vi "Begin.vi"(8 "error in":errorcluster) -> (0 "error out":errorcluster)   [LabVIEW 2019]
doc: "Called before other user functions, this VI is expected to open initial I/O refnums, load in file data, and do all program initialization. Notice that the <B>error out</B> terminal is simply used for data flow. Wiring it to other structures or subVIs ensures that this VI runs first."
uses:
  <vilib>/Rock Robotics/WPI/DriverStation/WPI_DriverStationRobotMode2.ctl
  <vilib>/Rock Robotics/WPI/Joystick/WPI_JoystickDeviceEnum.ctl
  <vilib>/Rock Robotics/SystemInterfaces/DIO/FPGA_DIOChannel.ctl
  <vilib>/Rock Robotics/WPI/ThirdParty/REV Robotics/SPARK MAX/Typedef/Spark MAX Idle Mode.ctl
  <vilib>/Rock Robotics/WPI/ThirdParty/REV Robotics/SPARK MAX/Typedef/Spark MAX Motor Type.ctl
  <vilib>/Rock Robotics/WPI/SafetyOutput/WPI_SafetyOutputConfigMenu.ctl
  <vilib>/Rock Robotics/WPI/Solenoid/WPI_SolenoidChannel.ctl
  <vilib>/Rock Robotics/WPI/Encoder/WPI_EncoderType.ctl
  <vilib>/Rock Robotics/SystemInterfaces/DIO/FPGA_DIORelayChannel.ctl
  <vilib>/Rock Robotics/WPI/Relay/WPI_RelayDirection.ctl
  <vilib>/Rock Robotics/WPI/ThirdParty/Phoenix-LabVIEW/Motor Controller/Controls/CTRE_Phoenix_MotorControl_ControlMode.ctl
  Robot Global Data.vi
  <vilib>/Rock Robotics/Network Tables/NT Write String Array.vi
  <vilib>/Rock Robotics/WPI/Counter/WPI_CounterDigitalInputToDigitalSource.vi
  <vilib>/Rock Robotics/WPI/RobotDrive/WPI_RobotDriveOpen4MotorWithExistingMotors.vi
  <vilib>/Rock Robotics/WPI/Solenoid/WPI_SolenoidOpenDouble.vi
  <vilib>/Rock Robotics/WPI/Switch/WPI_SwitchOpenLimit.vi
  <vilib>/Rock Robotics/WPI/Utilities/WPI_GetSetVariantRefNum.vi
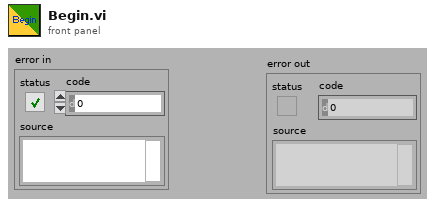
[diagram p1: front panel]
types:
  T1 = typedef "CTRE_Phoenix_MotorControl_ControlMode.ctl" = u16
  T2 = typedef "WPI_RelayDirection.ctl" = enum16{"Both directions", "Forward only", "Reverse only"}
  T3 = typedef "FPGA_DIORelayChannel.ctl" = enum8{"Relay 0", "Relay 1", "Relay 2", "Relay 3", "Invalid"}
  T4 = typedef "WPI_SolenoidChannel.ctl" = enum8{"Solenoid 0", "Solenoid 1", "Solenoid 2", "Solenoid 3", "Solenoid 4", "Solenoid 5", "Solenoid 6", "Solenoid 7", "Invalid"}
  T5 = typedef "WPI_EncoderType.ctl" = enum16{"1x", "2x", "4x"}
  T6 = typedef "FPGA_DIOChannel.ctl" = enum8{"DIO 0", "DIO 1", "DIO 2", "DIO 3", "DIO 4", "DIO 5", "DIO 6", "DIO 7", "DIO 8", "DIO 9", "DIO MXP 0", "DIO MXP 1", "DIO MXP 2", "DIO MXP 3", "DIO MXP 4", "DIO MXP 5", "DIO MXP 6", "DIO MXP 7", "DIO MXP 8", "DIO MXP 9", "DIO MXP 10", "DIO MXP 11", "DIO MXP 12", "DIO MXP 13", "DIO MXP 14", "DIO MXP 15", "SPI Port CS1", "SPI Port CS2", "SPI Port CS3", "SPI Port MISO", "SPI Port MOSI", "Invalid"}
  T7 = typedef "WPI_SafetyOutputConfigMenu.ctl" = enum16{"Enable", "Disable"}
  T8 = typedef "Spark MAX Idle Mode.ctl" = enum16{"Coast", "Brake"}
  T9 = typedef "Spark MAX Motor Type.ctl" = enum16{"Brushed", "Brushless"}
  T10 = typedef "WPI_JoystickDeviceEnum.ctl" = enum16{"USB 0", "USB 1", "USB 2", "USB 3", "USB 4", "USB 5"}
  T11 = typedef "WPI_DriverStationRobotMode2.ctl" = enum16{"Autonomous Disabled", "Autonomous Enabled", "Teleop Disabled", "Teleop Enabled", "Disconnected", "Finish", "Test Disabled", "Test Enabled", "Emergency Stopped"}
  T12 = typedef "WPI_MotorControlDeviceRef.ctl" = cluster{"DeviceStatus":errorcluster, "Type":T13, "PWM":cluster{"PWM Channel":T14, "DeadBand":T15}, "CAN":cluster{"Device Number":u8, "SetOutput VI Ref":variant, "GetOutput VI Ref":variant, "Enable VI Ref":variant, "Disable VI Ref":variant, "Data":variant}, "Invert":bool, "DIO PWM":cluster{"PWM \"Enable\" Channel":T14, "DIOChannel":T6, "PWM Rate":dbl}}
  T13 = typedef "WPI_MotorControlType.ctl" = enum16{"PWM", "CAN", "DIO PWM"}
  T14 = typedef "FPGA_DIOPWMChannel.ctl" = enum8{"PWM 0", "PWM 1", "PWM 2", "PWM 3", "PWM 4", "PWM 5", "PWM 6", "PWM 7", "PWM 8", "PWM 9", "PWM MXP 0", "PWM MXP 1", "PWM MXP 2", "PWM MXP 3", "PWM MXP 4", "PWM MXP 5", "PWM MXP 6", "PWM MXP 7", "PWM MXP 8", "PWM MXP 9", "Invalid"}
  T15 = typedef "WPI_PWMDeadband.ctl" = cluster{"Name":string, "maxPositivePwm":i32, "minPositivePwm":i32, "centerPwm":i32, "maxNegativePwm":i32, "minNegativePwm":i32, "angularRange":u16}
  T16 = typedef "WPI_JoystickDevRef.ctl" = cluster{"Device":T10}
  T17 = typedef "WPI_RobotDriveDevRef.ctl" = cluster{"DevStatus":errorcluster, "Motors[]":T12[], "Square Inputs":bool, "Max Output":dbl}
  T18 = typedef "WPI_SolenoidDevRef.ctl" = cluster{"DevStatus":errorcluster, "Pneumatics Control Module":u8, "Forward Solenoid Channel":T4, "Reverse Solenoid Channel":T4}
  T19 = typedef "WPI_DigitalInputDevRef.ctl" = cluster{"DevStatus":errorcluster, "DIO Channel":T6}
  T20 = typedef "FPGA_CounterEncoderSourceConvertionLVSourceType.ctl" = cluster{"DevStatus":errorcluster, "AnalogTriggerMode?":bool, "DigitalMode":cluster{"DIO Channel":T21}, "AnalogTriggerMode":cluster{"AnalogTriggerIndex":T22, "OutputType":T23}}
  T21 = typedef "FPGA_DIODigitalSourceChannel.ctl" = enum8{"DIO 0", "DIO 1", "DIO 2", "DIO 3", "DIO 4", "DIO 5", "DIO 6", "DIO 7", "DIO 8", "DIO 9", "DIO MXP 0", "DIO MXP 1", "DIO MXP 2", "DIO MXP 3", "DIO MXP 4", "DIO MXP 5", "DIO MXP 6", "DIO MXP 7", "DIO MXP 8", "DIO MXP 9", "DIO MXP 10", "DIO MXP 11", "DIO MXP 12", "DIO MXP 13", "DIO MXP 14", "DIO MXP 15", "SPI Port CS1", "SPI Port CS2", "SPI Port CS3", "SPI Port MISO", "SPI Port MOSI", "Disabled"}
  T22 = typedef "FPGA_AnalogTriggerIndex.ctl" = enum8{"Trig 0", "Trig 1", "Trig 2", "Trig 3", "Trig 4", "Trig 5", "Trig 6", "Trig 7", "Invalid"}
  T23 = typedef "FPGA_AnalogTriggerOutType.ctl" = enum16{"InWindow", "TriggerState", "Rising", "Falling"}
  T24 = typedef "WPI_EncoderDevRef.ctl" = cluster{"DevStatus":errorcluster, "EncoderIndex":T25, "CounterIndex":T26, "DistancePerCount":dbl, "Decoding Type":T5}
  T25 = typedef "FPGA_EncoderIdx.ctl" = enum8{"Enc 0", "Enc 1", "Enc 2", "Enc 3", "Enc 4", "Enc 5", "Enc 6", "Enc 7", "Invalid"}
  T26 = typedef "FPGA_CounterCtrSystemIndex.ctl" = enum8{"Ctr 0", "Ctr 1", "Ctr 2", "Ctr 3", "Ctr 4", "Ctr 5", "Ctr 6", "Ctr 7", "Invalid"}
  T27 = typedef "WPI_CompressorDevRef.ctl" = cluster{"DevStatus":errorcluster, "Pneumatics Control Module":u8}
  T28 = typedef "WPI_SwitchDevRef.ctl" = cluster{"DevStatus":errorcluster, "DIO Channel":T6, "CntIndex":T26, "Normally Closed":bool}
  T29 = typedef "WPI_RelayDevRef.ctl" = cluster{"DevStatus":errorcluster, "Relay Channel":T3, "Relay Direction":T2}
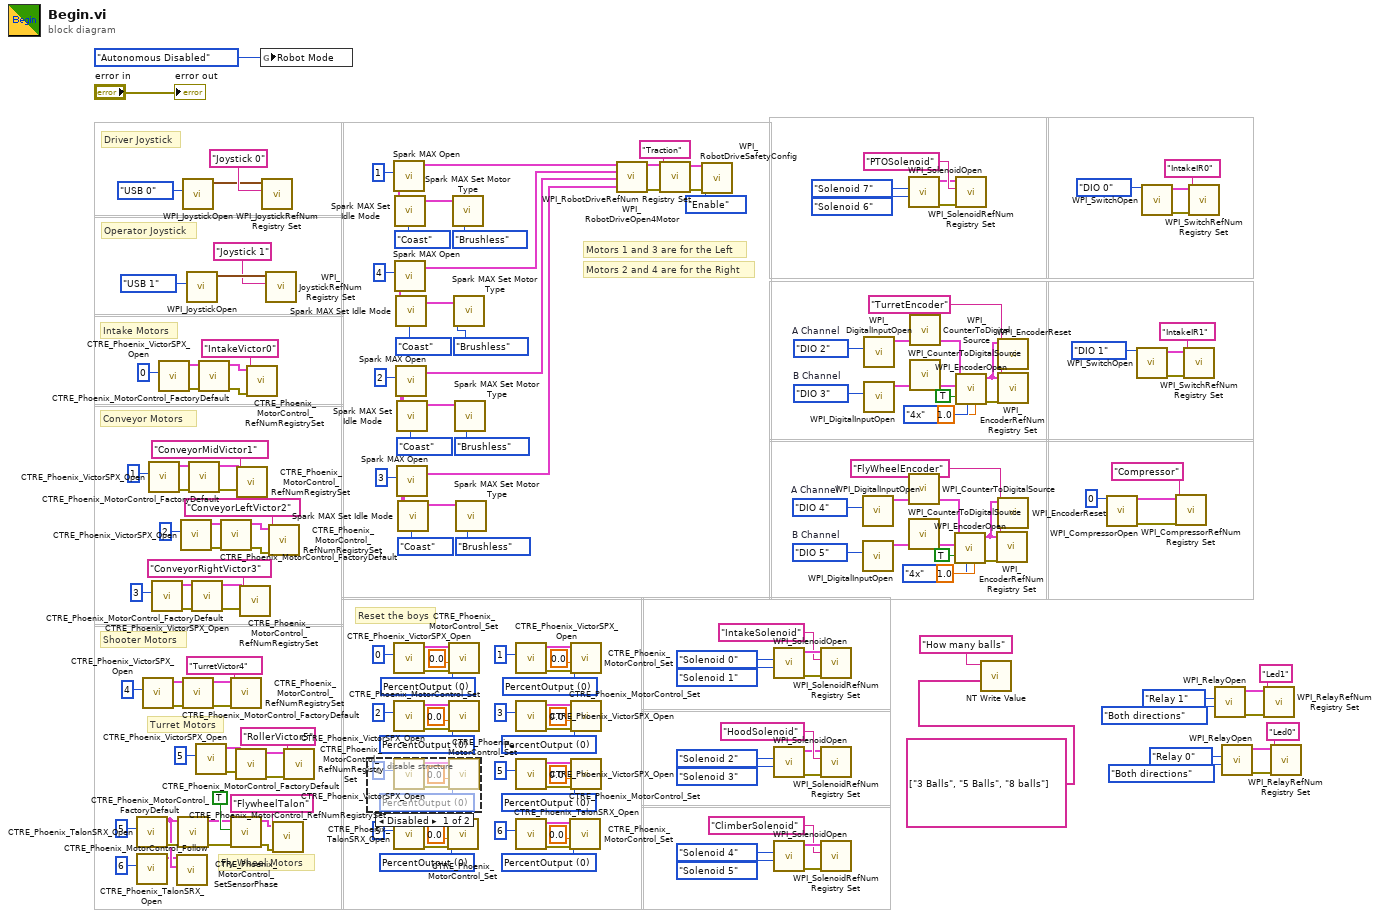
[diagram p0: block diagram]
diagram:
  w8 = T1 0 items=["PercentOutput"=0, "Position"=1, "Velocity"=2, "Current"=3, "Follower"=5, "MotionProfile"=6, "MotionMagic"=7, "MotionMagicArc"=8, "MotionProfileArc"=10, "Disabled"=15] ("Control Mode")
  w16 = T1 0 items=["PercentOutput"=0, "Position"=1, "Velocity"=2, "Current"=3, "Follower"=5, "MotionProfile"=6, "MotionMagic"=7, "MotionMagicArc"=8, "MotionProfileArc"=10, "Disabled"=15] ("Control Mode")
  w17 = T1 0 items=["PercentOutput"=0, "Position"=1, "Velocity"=2, "Current"=3, "Follower"=5, "MotionProfile"=6, "MotionMagic"=7, "MotionMagicArc"=8, "MotionProfileArc"=10, "Disabled"=15] ("Control Mode")
  w84 = FPGA_DIOChannel."DIO 3"  # B Channel
  w85 = FPGA_DIOChannel."DIO 2"  # A Channel
  w124 = T1 0 items=["PercentOutput"=0, "Position"=1, "Velocity"=2, "Current"=3, "Follower"=5, "MotionProfile"=6, "MotionMagic"=7, "MotionMagicArc"=8, "MotionProfileArc"=10, "Disabled"=15] ("Control Mode")
  w123 = T1 0 items=["PercentOutput"=0, "Position"=1, "Velocity"=2, "Current"=3, "Follower"=5, "MotionProfile"=6, "MotionMagic"=7, "MotionMagicArc"=8, "MotionProfileArc"=10, "Disabled"=15] ("Control Mode")
  w133 = T1 0 items=["PercentOutput"=0, "Position"=1, "Velocity"=2, "Current"=3, "Follower"=5, "MotionProfile"=6, "MotionMagic"=7, "MotionMagicArc"=8, "MotionProfileArc"=10, "Disabled"=15] ("Control Mode")
  w134 = T1 0 items=["PercentOutput"=0, "Position"=1, "Velocity"=2, "Current"=3, "Follower"=5, "MotionProfile"=6, "MotionMagic"=7, "MotionMagicArc"=8, "MotionProfileArc"=10, "Disabled"=15] ("Control Mode")
  w170 = FPGA_DIOChannel."DIO 5"  # B Channel
  w169 = FPGA_DIOChannel."DIO 4"  # A Channel
  # "Turret Motors"
  # "Fly Wheel Motors"
  # "Shooter Motors"
  # "Conveyor Motors"
  # "Intake Motors"
  # "Reset the boys"
  # "Motors 2 and 4 are for the Right"
  # "Motors 1 and 3 are for the Left"
  # "Operator Joystick"
  # "Driver Joystick"
  n1 = call <vilib>:"CTRE_Phoenix_TalonSRX_Open.vi"("Device Number"=u8 5) -> ("error out"=w31:errorcluster, "CAN Talon SRX Ref"=w30:T12)  [unwired: 9 in]
  n2 = call <vilib>:"CTRE_Phoenix_TalonSRX_Open.vi"("Device Number"=u8 6) -> ("CAN Talon SRX Ref"=w23:T12)  [unwired: 9 in, 1 out]
  n3 = call <vilib>:"CTRE_Phoenix_VictorSPX_Open.vi"("Device Number"=u8 4) -> ("error out"=w6:errorcluster, "CAN Talon SRX Ref"=w5:T12)  [unwired: 9 in]
  n4 = call <vilib>:"CTRE_Phoenix_VictorSPX_Open.vi"("Device Number"=u8 1) -> ("error out"=w51:errorcluster, "CAN Talon SRX Ref"=w52:T12)  [unwired: 9 in]
  n5 = call <vilib>:"CTRE_Phoenix_VictorSPX_Open.vi"("Device Number"=u8 3) -> ("error out"=w39:errorcluster, "CAN Talon SRX Ref"=w40:T12)  [unwired: 9 in]
  n6 = call <vilib>:"CTRE_Phoenix_VictorSPX_Open.vi"("Device Number"=u8 0) -> ("error out"=w62:errorcluster, "CAN Talon SRX Ref"=w61:T12)  [unwired: 9 in]
  n7 = call <vilib>:"CTRE_Phoenix_MotorControl_Follow.vi"("Master Controller to Follow"=w30, "PhoenixMotorControlDevRef"=w23) -> ()  [unwired: 8 in, 2 out]
  n8 = call <vilib>:"CTRE_Phoenix_MotorControl_FactoryDefault.vi"("error in"=w31, "PhoenixMotorControlDevRef"=w30) -> ("error out"=w34:errorcluster, "PhoenixMotorControlDevRef"=w35:T12)  [unwired: 8 in]
  n9 = call <vilib>:"CTRE_Phoenix_VictorSPX_Open.vi"("Device Number"=u8 2) -> ("error out"=w50:errorcluster, "CAN Talon SRX Ref"=w49:T12)  [unwired: 9 in]
  n10 = call <vilib>:"WPI_JoystickOpen.vi"("JoystickDevice"=WPI_JoystickDeviceEnum."USB 0") -> ("JoystickDevRef"=w178:T16)  [unwired: 10 in]
  n11 = call <vilib>:"CTRE_Phoenix_MotorControl_FactoryDefault.vi"("error in"=w6, "PhoenixMotorControlDevRef"=w5) -> ("error out"=w4:errorcluster, "PhoenixMotorControlDevRef"=w2:T12)  [unwired: 8 in]
  n12 = call <vilib>:"WPI_JoystickOpen.vi"("JoystickDevice"=WPI_JoystickDeviceEnum."USB 1") -> ("JoystickDevRef"=w173:T16)  [unwired: 10 in]
  n13 = call <vilib>:"CTRE_Phoenix_MotorControl_FactoryDefault.vi"("error in"=w51, "PhoenixMotorControlDevRef"=w52) -> ("error out"=w53:errorcluster, "PhoenixMotorControlDevRef"=w54:T12)  [unwired: 8 in]
  n14 = call <vilib>:"CTRE_Phoenix_MotorControl_FactoryDefault.vi"("error in"=w39, "PhoenixMotorControlDevRef"=w40) -> ("error out"=w41:errorcluster, "PhoenixMotorControlDevRef"=w42:T12)  [unwired: 8 in]
  n15 = call <vilib>:"CTRE_Phoenix_VictorSPX_Open.vi"("Device Number"=u8 5) -> ("error out"=w24:errorcluster, "CAN Talon SRX Ref"=w25:T12)  [unwired: 9 in]
  n16 = call <vilib>:"CTRE_Phoenix_MotorControl_FactoryDefault.vi"("error in"=w62, "PhoenixMotorControlDevRef"=w61) -> ("error out"=w60:errorcluster, "PhoenixMotorControlDevRef"=w59:T12)  [unwired: 8 in]
  n17 = call <vilib>:"CTRE_Phoenix_MotorControl_FactoryDefault.vi"("error in"=w50, "PhoenixMotorControlDevRef"=w49) -> ("error out"=w48:errorcluster, "PhoenixMotorControlDevRef"=w47:T12)  [unwired: 8 in]
  n18 = call <vilib>:"CTRE_Phoenix_MotorControl_RefNumRegistrySet.vi"("error in (no error)"=w4, "refnum name"="TurretVictor4", "PhoenixMotorControlDevRef"=w2) -> ()  [unwired: 7 in, 2 out]
  n19 = call <vilib>:"CTRE_Phoenix_MotorControl_SetSensorPhase.vi"("error in (no error)"=w34, "PhaseSensor"=TRUE, "PhoenixMotorControlDevRef"=w35) -> ("error out"=w32:errorcluster, "PhoenixMotorControlDevRef"=w33:T12)  [unwired: 7 in]
  n20 = call <vilib>:"CTRE_Phoenix_MotorControl_FactoryDefault.vi"("error in"=w24, "PhoenixMotorControlDevRef"=w25) -> ("error out"=w26:errorcluster, "PhoenixMotorControlDevRef"=w28:T12)  [unwired: 8 in]
  n21 = call <vilib>:"CTRE_Phoenix_MotorControl_RefNumRegistrySet.vi"("error in (no error)"=w53, "refnum name"="ConveyorMidVictor1", "PhoenixMotorControlDevRef"=w54) -> ()  [unwired: 7 in, 2 out]
  n22 = call <vilib>:"CTRE_Phoenix_MotorControl_RefNumRegistrySet.vi"("error in (no error)"=w41, "refnum name"="ConveyorRightVictor3", "PhoenixMotorControlDevRef"=w42) -> ()  [unwired: 7 in, 2 out]
  n23 = call <vilib>:"CTRE_Phoenix_MotorControl_RefNumRegistrySet.vi"("error in (no error)"=w60, "refnum name"="IntakeVictor0", "PhoenixMotorControlDevRef"=w59) -> ()  [unwired: 7 in, 2 out]
  n24 = global write "Robot Global Data.vi" "Robot Mode"(WPI_DriverStationRobotMode2."Autonomous Disabled" ("Robot Mode")) -> ()
  n25 = call <vilib>:"WPI_JoystickRefNum Registry Set.vi"("refnum name"="Joystick 0", "JoystickDevRef"=w178) -> ()  [unwired: 8 in, 2 out]
  n26 = call <vilib>:"WPI_JoystickRefNum Registry Set.vi"("refnum name"="Joystick 1", "JoystickDevRef"=w173) -> ()  [unwired: 8 in, 2 out]
  n27 = call <vilib>:"CTRE_Phoenix_MotorControl_RefNumRegistrySet.vi"("error in (no error)"=w48, "refnum name"="ConveyorLeftVictor2", "PhoenixMotorControlDevRef"=w47) -> ()  [unwired: 7 in, 2 out]
  n28 = call <vilib>:"CTRE_Phoenix_MotorControl_RefNumRegistrySet.vi"("error in (no error)"=w32, "refnum name"="FlywheelTalon", "PhoenixMotorControlDevRef"=w33) -> ()  [unwired: 7 in, 2 out]
  n29 = call <vilib>:"CTRE_Phoenix_MotorControl_RefNumRegistrySet.vi"("error in (no error)"=w26, "refnum name"="RollerVictor5", "PhoenixMotorControlDevRef"=w28) -> ()  [unwired: 7 in, 2 out]
  n30 = disable-structure shown="Disabled" {
    frame Disabled {
      w185 = T1 0 items=["PercentOutput"=0, "Position"=1, "Velocity"=2, "Current"=3, "Follower"=5, "MotionProfile"=6, "MotionMagic"=7, "MotionMagicArc"=8, "MotionProfileArc"=10, "Disabled"=15] ("Control Mode")
      n31 = call <vilib>:"CTRE_Phoenix_VictorSPX_Open.vi"("Device Number"=u8 4) -> ("error out"=w181:errorcluster, "CAN Talon SRX Ref"=w182:T12)  [unwired: 9 in]
      n32 = call <vilib>:"CTRE_Phoenix_MotorControl_Set.vi"("error in (no error)"=w181, "Output"=0.0, "Control Mode"=w185, "PhoenixMotorControlDevRef"=w182) -> ()  [unwired: 6 in, 2 out]
    }
    frame Enabled {
    }
  }
  n33 = call <vilib>:"Spark MAX Open.vi"("Device Number"=u8 1) -> ("MotorControlDeviceRef"=w157:T12)  [unwired: 9 in, 1 out]
  n34 = call <vilib>:"CTRE_Phoenix_VictorSPX_Open.vi"("Device Number"=u8 0) -> ("error out"=w138:errorcluster, "CAN Talon SRX Ref"=w137:T12)  [unwired: 9 in]
  n35 = call <vilib>:"CTRE_Phoenix_VictorSPX_Open.vi"("Device Number"=u8 2) -> ("error out"=w129:errorcluster, "CAN Talon SRX Ref"=w130:T12)  [unwired: 9 in]
  n36 = call <vilib>:"CTRE_Phoenix_TalonSRX_Open.vi"("Device Number"=u8 5) -> ("error out"=w21:errorcluster, "CAN Talon SRX Ref"=w20:T12)  [unwired: 9 in]
  n37 = call <vilib>:"Spark MAX Set Idle Mode.vi"("Idle Mode"=Spark_MAX_Idle_Mode."Coast", "MotorControlDeviceRef in"=w157) -> ()  [unwired: 8 in, 2 out]
  n38 = call <vilib>:"Spark MAX Open.vi"("Device Number"=u8 4) -> ("MotorControlDeviceRef"=w153:T12)  [unwired: 9 in, 1 out]
  n39 = call <vilib>:"Spark MAX Set Idle Mode.vi"("Idle Mode"=Spark_MAX_Idle_Mode."Coast", "MotorControlDeviceRef in"=w153) -> ()  [unwired: 8 in, 2 out]
  n40 = call <vilib>:"Spark MAX Open.vi"("Device Number"=u8 2) -> ("MotorControlDeviceRef"=w149:T12)  [unwired: 9 in, 1 out]
  n41 = call <vilib>:"Spark MAX Set Idle Mode.vi"("Idle Mode"=Spark_MAX_Idle_Mode."Coast", "MotorControlDeviceRef in"=w149) -> ()  [unwired: 8 in, 2 out]
  n42 = call <vilib>:"Spark MAX Open.vi"("Device Number"=u8 3) -> ("MotorControlDeviceRef"=w145:T12)  [unwired: 9 in, 1 out]
  n43 = call <vilib>:"Spark MAX Set Idle Mode.vi"("Idle Mode"=Spark_MAX_Idle_Mode."Coast", "MotorControlDeviceRef in"=w145) -> ()  [unwired: 8 in, 2 out]
  n44 = call <vilib>:"CTRE_Phoenix_MotorControl_Set.vi"("error in (no error)"=w21, "Output"=0.0, "Control Mode"=w17, "PhoenixMotorControlDevRef"=w20) -> ()  [unwired: 6 in, 2 out]
  n45 = call <vilib>:"CTRE_Phoenix_MotorControl_Set.vi"("error in (no error)"=w138, "Output"=0.0, "Control Mode"=w134, "PhoenixMotorControlDevRef"=w137) -> ()  [unwired: 6 in, 2 out]
  n46 = call <vilib>:"CTRE_Phoenix_MotorControl_Set.vi"("error in (no error)"=w129, "Output"=0.0, "Control Mode"=w133, "PhoenixMotorControlDevRef"=w130) -> ()  [unwired: 6 in, 2 out]
  n47 = call <vilib>:"Spark MAX Set Motor Type.vi"("Motor Type"=Spark_MAX_Motor_Type."Brushless", "MotorControlDevRef"=w157) -> ()  [unwired: 8 in, 2 out]
  n48 = call <vilib>:"Spark MAX Set Motor Type.vi"("Motor Type"=Spark_MAX_Motor_Type."Brushless", "MotorControlDevRef"=w153) -> ()  [unwired: 8 in, 2 out]
  n49 = call <vilib>:"Spark MAX Set Motor Type.vi"("Motor Type"=Spark_MAX_Motor_Type."Brushless", "MotorControlDevRef"=w149) -> ()  [unwired: 8 in, 2 out]
  n50 = call <vilib>:"Spark MAX Set Motor Type.vi"("Motor Type"=Spark_MAX_Motor_Type."Brushless", "MotorControlDevRef"=w145) -> ()  [unwired: 8 in, 2 out]
  n51 = call <vilib>:"CTRE_Phoenix_VictorSPX_Open.vi"("Device Number"=u8 1) -> ("error out"=w119:errorcluster, "CAN Talon SRX Ref"=w120:T12)  [unwired: 9 in]
  n52 = call <vilib>:"CTRE_Phoenix_VictorSPX_Open.vi"("Device Number"=u8 3) -> ("error out"=w128:errorcluster, "CAN Talon SRX Ref"=w127:T12)  [unwired: 9 in]
  n53 = call <vilib>:"CTRE_Phoenix_VictorSPX_Open.vi"("Device Number"=u8 5) -> ("error out"=w11:errorcluster, "CAN Talon SRX Ref"=w7:T12)  [unwired: 9 in]
  n54 = call <vilib>:"CTRE_Phoenix_TalonSRX_Open.vi"("Device Number"=u8 6) -> ("error out"=w12:errorcluster, "CAN Talon SRX Ref"=w13:T12)  [unwired: 9 in]
  n55 = call <vilib>:"CTRE_Phoenix_MotorControl_Set.vi"("error in (no error)"=w12, "Output"=0.0, "Control Mode"=w16, "PhoenixMotorControlDevRef"=w13) -> ()  [unwired: 6 in, 2 out]
  n56 = call <vilib>:"CTRE_Phoenix_MotorControl_Set.vi"("error in (no error)"=w119, "Output"=0.0, "Control Mode"=w123, "PhoenixMotorControlDevRef"=w120) -> ()  [unwired: 6 in, 2 out]
  n57 = call <vilib>:"CTRE_Phoenix_MotorControl_Set.vi"("error in (no error)"=w128, "Output"=0.0, "Control Mode"=w124, "PhoenixMotorControlDevRef"=w127) -> ()  [unwired: 6 in, 2 out]
  n58 = call <vilib>:"CTRE_Phoenix_MotorControl_Set.vi"("error in (no error)"=w11, "Output"=0.0, "Control Mode"=w8, "PhoenixMotorControlDevRef"=w7) -> ()  [unwired: 6 in, 2 out]
  n59 = call-poly <vilib>:"WPI_RobotDriveOpen4Motor.vi"("Rear Left Motor Dev Ref"=w157, "Rear Right Motor Dev Ref"=w153, "Front Left Motor Dev Ref"=w149, "Front Right Motor Dev Ref"=w145) -> ("RobotDriveDevRef"=w143:T17, "error out"=w144:errorcluster)  [unwired: 10 in]
  n60 = call <vilib>:"WPI_RobotDriveRefNum Registry Set.vi"("error in (no error)"=w144, "refnum name"="Traction", "RobotDriveDevRef"=w143) -> ("error out"=w141:errorcluster, "RobotDriveDevRef"=w140:T17)  [unwired: 7 in]
  n61 = call <vilib>:"WPI_RobotDriveSafetyConfig.vi"("error in (no error)"=w141, "mode"=WPI_SafetyOutputConfigMenu."Enable", "RobotDriveDevRef"=w140) -> ()  [unwired: 7 in, 2 out]
  n62 = call-poly <vilib>:"WPI_SolenoidOpen.vi"("Reverse Solenoid Channel"=WPI_SolenoidChannel."Solenoid 1", "Forward Solenoid Channel"=WPI_SolenoidChannel."Solenoid 0") -> ("error out"=w118:errorcluster, "SolenoidDevRef"=w117:T18)  [unwired: 8 in]
  n63 = call-poly <vilib>:"WPI_SolenoidOpen.vi"("Reverse Solenoid Channel"=WPI_SolenoidChannel."Solenoid 3", "Forward Solenoid Channel"=WPI_SolenoidChannel."Solenoid 2") -> ("error out"=w109:errorcluster, "SolenoidDevRef"=w110:T18)  [unwired: 8 in]
  n64 = call-poly <vilib>:"WPI_SolenoidOpen.vi"("Reverse Solenoid Channel"=WPI_SolenoidChannel."Solenoid 5", "Forward Solenoid Channel"=WPI_SolenoidChannel."Solenoid 4") -> ("error out"=w108:errorcluster, "SolenoidDevRef"=w107:T18)  [unwired: 8 in]
  n65 = call <vilib>:"WPI_SolenoidRefNum Registry Set.vi"("error in (no error)"=w118, "refnum name"="IntakeSolenoid", "SolenoidDevRef"=w117) -> ()  [unwired: 7 in, 2 out]
  n66 = call <vilib>:"WPI_SolenoidRefNum Registry Set.vi"("error in (no error)"=w109, "refnum name"="HoodSolenoid", "SolenoidDevRef"=w110) -> ()  [unwired: 7 in, 2 out]
  n67 = call <vilib>:"WPI_SolenoidRefNum Registry Set.vi"("error in (no error)"=w108, "refnum name"="ClimberSolenoid", "SolenoidDevRef"=w107) -> ()  [unwired: 7 in, 2 out]
  n68 = call <vilib>:"WPI_DigitalInputOpen.vi"("DIO Channel"=w169) -> ("DigitalInputDevRef"=w166:T19)  [unwired: 1 in, 9 out]
  n69 = call <vilib>:"WPI_DigitalInputOpen.vi"("DIO Channel"=w170) -> ("DigitalInputDevRef"=w167:T19)  [unwired: 1 in, 9 out]
  n70 = call <vilib>:"WPI_DigitalInputOpen.vi"("DIO Channel"=w85) -> ("DigitalInputDevRef"=w88:T19)  [unwired: 1 in, 9 out]
  n71 = call <vilib>:"WPI_DigitalInputOpen.vi"("DIO Channel"=w84) -> ("DigitalInputDevRef"=w87:T19)  [unwired: 1 in, 9 out]
  n72 = call-poly <vilib>:"WPI_SolenoidOpen.vi"("Reverse Solenoid Channel"=WPI_SolenoidChannel."Solenoid 6", "Forward Solenoid Channel"=WPI_SolenoidChannel."Solenoid 7") -> ("error out"=w77:errorcluster, "SolenoidDevRef"=w78:T18)  [unwired: 8 in]
  n73 = call-poly <vilib>:"WPI_CounterToDigitalSource.vi"("DigitalInputDevRef"=w166) -> ("Digital Source"=w165:T20)  [unwired: 6 out]
  n74 = call-poly <vilib>:"WPI_CounterToDigitalSource.vi"("DigitalInputDevRef"=w167) -> ("Digital Source"=w168:T20)  [unwired: 6 out]
  n75 = call-poly <vilib>:"WPI_CounterToDigitalSource.vi"("DigitalInputDevRef"=w88) -> ("Digital Source"=w89:T20)  [unwired: 6 out]
  n76 = call-poly <vilib>:"WPI_CounterToDigitalSource.vi"("DigitalInputDevRef"=w87) -> ("Digital Source"=w86:T20)  [unwired: 6 out]
  n77 = call <vilib>:"WPI_EncoderOpen.vi"("DistancePerCount"=1.0, "Decoding Type"=WPI_EncoderType."4x", "Invert Direction (False)"=TRUE, "BSource"=w168, "ASource"=w165) -> ("error out"=w162:errorcluster, "EncoderDevRef"=w94:T24)  [unwired: 3 in, 2 out]
  n78 = call <vilib>:"WPI_SolenoidRefNum Registry Set.vi"("error in (no error)"=w77, "refnum name"="PTOSolenoid", "SolenoidDevRef"=w78) -> ()  [unwired: 7 in, 2 out]
  n79 = call <vilib>:"WPI_EncoderOpen.vi"("DistancePerCount"=1.0, "Decoding Type"=WPI_EncoderType."4x", "Invert Direction (False)"=TRUE, "BSource"=w86, "ASource"=w89) -> ("error out"=w92:errorcluster, "EncoderDevRef"=w82:T24)  [unwired: 3 in, 2 out]
  n80 = call-poly <vilib>:"NT Write Value.vi"("String Array"=string[] ["3 Balls", "5 Balls", "8 balls"], "Name"="How many balls") -> ()  [unwired: 9 in, 1 out]
  n81 = call <vilib>:"WPI_EncoderRefNum Registry Set.vi"("error in (no error)"=w162, "refnum name"="FlyWheelEncoder", "EncoderDevRef"=w94) -> ()  [unwired: 7 in, 2 out]
  n82 = call <vilib>:"WPI_EncoderReset.vi"("EncoderDevRef"=w82) -> ()  [unwired: 9 in, 2 out]
  n83 = call <vilib>:"WPI_EncoderRefNum Registry Set.vi"("error in (no error)"=w92, "refnum name"="TurretEncoder", "EncoderDevRef"=w82) -> ()  [unwired: 7 in, 2 out]
  n84 = call <vilib>:"WPI_EncoderReset.vi"("EncoderDevRef"=w94) -> ()  [unwired: 9 in, 2 out]
  n85 = call <vilib>:"WPI_CompressorOpen.vi"("Pneumatics Control Module (0)"=u8 0) -> ("CompressorDevRef"=w76:T27, "error out"=w75:errorcluster)  [unwired: 13 in]
  n86 = call-poly <vilib>:"WPI_SwitchOpen.vi"("DIO Channel"=FPGA_DIOChannel."DIO 1") -> ("error out"=w96:errorcluster, "SwitchDevRef"=w97:T28)  [unwired: 9 in]
  n87 = call-poly <vilib>:"WPI_SwitchOpen.vi"("DIO Channel"=FPGA_DIOChannel."DIO 0") -> ("error out"=w101:errorcluster, "SwitchDevRef"=w100:T28)  [unwired: 9 in]
  n88 = call <vilib>:"WPI_CompressorRefNum Registry Set.vi"("error in (no error)"=w75, "refnum name"="Compressor", "CompressorDevRef"=w76) -> ()  [unwired: 7 in, 2 out]
  n89 = call <vilib>:"WPI_SwitchRefNum Registry Set.vi"("error in (no error)"=w96, "refnum name"="IntakeIR1", "SwitchDevRef"=w97) -> ()  [unwired: 7 in, 2 out]
  n90 = call <vilib>:"WPI_SwitchRefNum Registry Set.vi"("error in (no error)"=w101, "refnum name"="IntakeIR0", "SwitchDevRef"=w100) -> ()  [unwired: 7 in, 2 out]
  n91 = call <vilib>:"WPI_RelayOpen.vi"("Relay Direction"=WPI_RelayDirection."Both directions", "Relay Channel"=FPGA_DIORelayChannel."Relay 1") -> ("error out"=w71:errorcluster, "RelayDevRef"=w72:T29)  [unwired: 8 in]
  n92 = call <vilib>:"WPI_RelayOpen.vi"("Relay Direction"=WPI_RelayDirection."Both directions", "Relay Channel"=FPGA_DIORelayChannel."Relay 0") -> ("error out"=w64:errorcluster, "RelayDevRef"=w63:T29)  [unwired: 8 in]
  n93 = call <vilib>:"WPI_RelayRefNum Registry Set.vi"("error in (no error)"=w71, "refnum name"="Led1", "RelayDevRef"=w72) -> ()  [unwired: 7 in, 2 out]
  n94 = call <vilib>:"WPI_RelayRefNum Registry Set.vi"("error in (no error)"=w64, "refnum name"="Led0", "RelayDevRef"=w63) -> ()  [unwired: 7 in, 2 out]
  "error out" <- "error in"
